vi "Find Relevant Stat Row.vi"(0 "Last Data Row":i32, 5 "Last Stat Row":i32, 7 "Data IDs":string[](array[string]), 9 "Stat IDs":string[](array[string]), 11 "Stat SelStart":i32) -> (4 "Data Row":i32, 15 "Stat Row":i32)   [LabVIEW 2013]
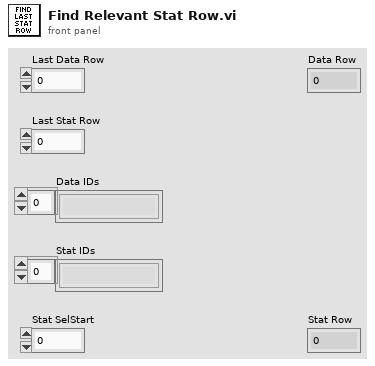
[diagram p1: front panel]
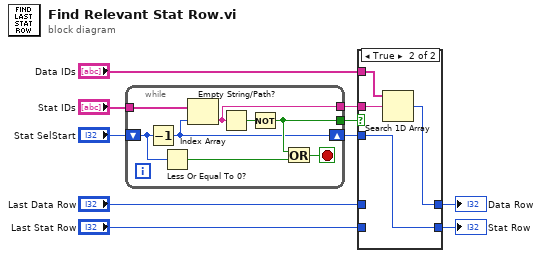
[diagram p0: block diagram]
diagram:
  n1 = while {
    tunnel: "Stat IDs" -> [w18]
    shift-right: [w12] -> w3
    shift-left: "Stat SelStart" -> [w17]
    tunnel: [w13] -> w8
    tunnel: [w11] -> w1
    stop <- w15 stop-if-true
    n2 = Decrement(x=w17) -> (x-1=w12:i32)
    n3 = Less Or Equal To 0?(x=w17) -> (x <= 0?=w16:bool)
    n4 = Index Array(array=w18, index=w12) -> (element=w11:string)
    n5 = Empty String/Path?(string/path=w11) -> (empty?=w14:bool)
    n6 = Not(x=w14) -> (.not. x?=w13:bool)
    n7 = Or(x=w13, y=w16) -> (x .or. y?=w15:bool)
  }
  n8 = case shown="True" w8 {
    tunnel: "Last Data Row" -> [w20 _]
    tunnel: "Last Stat Row" -> [w19 _]
    tunnel: [w20 w21] -> w5
    tunnel: [w19 w24] -> w4
    tunnel: w3 -> [_ w24]
    tunnel: "Data IDs" -> [_ w23]
    tunnel: w1 -> [_ w22]
    frame False {
    }
    frame True {
      n9 = Search 1D Array(1D array=w23, element=w22) -> (index of element=w21:i32)  [unwired: 1 in]
    }
  }
  "Data Row" <- w5
  "Stat Row" <- w4
